vi "io_query_long_data.vi"(4 "Simulation read buffer (\"Simulation\")":string="Simulation", 6 "Block Logging (F)":bool, 8 "error in":errorcluster, 9 "Max chunk read bytes count (65536)":u32=65536, 10 "write buffer":string, 11 "VISA resource name":refnum<visa-resource-name>) -> (0 "error out":errorcluster, 2 "read buffer":string, 3 "VISA resource name out":refnum<visa-resource-name>)   [LabVIEW 2014, in "rszvl_rsidr_core.lvlib"]
uses:
  rszvl_rsidr_core.lvlib
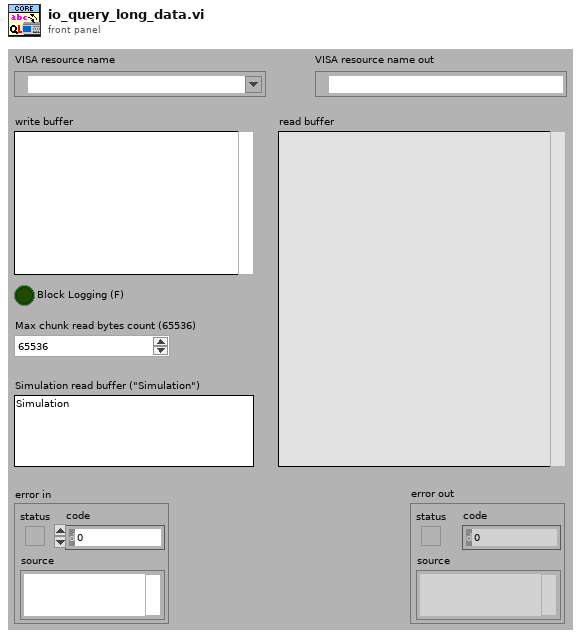
[diagram p1: front panel]
types:
  T1 = typedef "rszvl_rsidr_core.lvlib/type_Session_Data.ctl" = cluster{"Instr type":string, "Instr type for err. msg.":string, "Installed Options":string[], "OPC Timeout":i32, "Query Instrument Status":bool, "Check Range":bool, "Check Options":bool, "Add LF to Write":bool, "Simulate":bool, "Logging":bool, "Logging params":variant, "Interface Type":enum16{"Unknown", "GPIB", "VXI", "GPIB_VXI", "ASRL", "PXI", "TCPIP", "USB", "SOCKET"}, "Fast Sweep":i32, "AdditionalFlags":i32, "WaitBeforeWrite":i32, "WaitBeforeRead":i32, "BinDataChunkSize":i64}
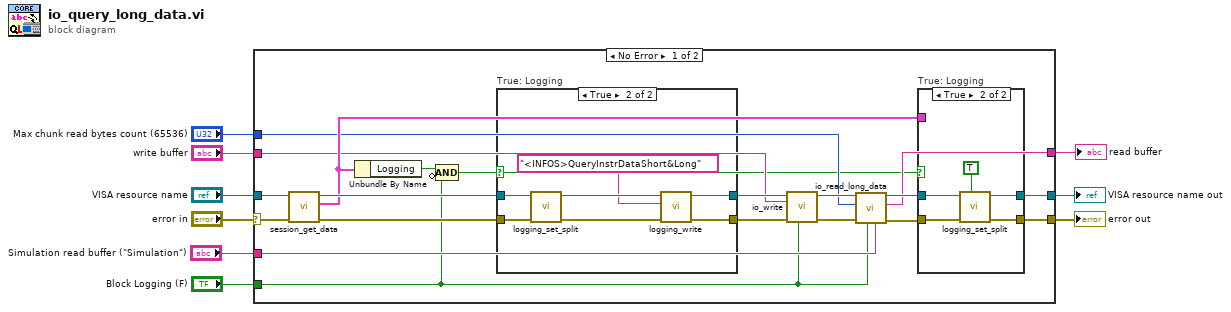
[diagram p0: block diagram]
diagram:
  n1 = case shown="No Error" "error in" {
    selector: "error in" -> [w19 w47]
    tunnel: [w13 w46] -> w3
    tunnel: [w14 w47] -> w2
    tunnel: "write buffer" -> [w16 _]
    tunnel: "VISA resource name" -> [w20 w46]
    tunnel: "Max chunk read bytes count (65536)" -> [w15 _]
    tunnel: "Simulation read buffer (\"Simulation\")" -> [w17 _]
    tunnel: [w18 _] -> w4
    tunnel: "Block Logging (F)" -> [w11 _]
    frame No Error {
      n2 = call "session_get_data.vi"("error in"=w19, "VISA resource name"=w20) -> ("error out"=w25:errorcluster, "Session User Data out"=w21:T1, "VISA resource name out"=w24:refnum<visa-resource-name>)  [unwired: 7 in]
      n3 = Unbundle By Name(w21) -> ("Logging"=w10:bool)
      n4 = Compound Arithmetic op=AND(w10, invert w11) -> (w12:bool)
      n5 = case "True: Logging" shown="True" w12 {
        tunnel: w25 -> [w38 w43]
        tunnel: w24 -> [w37 w42]
        tunnel: [w38 w45] -> w26
        tunnel: [w37 w44] -> w27
        frame False {
        }
        frame True {
          n6 = call "logging_set_split.vi"("error in"=w43, "VISA resource name"=w42) -> ("error out"=w41:errorcluster, "VISA resource name out"=w40:refnum<visa-resource-name>)  [unwired: 8 in]
          n7 = call "logging_write.vi"("error in"=w41, "String to write"="<INFOS>QueryInstrDataShort&Long" ("format string"), "VISA resource name"=w40) -> ("error out"=w45:errorcluster, "VISA resource name out"=w44:refnum<visa-resource-name>)  [unwired: 7 in]
        }
      }
      n8 = call "io_write.vi"("Block Logging (F)"=w11, "error in"=w26, "write buffer"=w16, "VISA resource name"=w27) -> ("error out"=w28:errorcluster, "VISA resource name out"=w29:refnum<visa-resource-name>)  [unwired: 6 in]
      n9 = call "io_read_long_data.vi"("Simulation read buffer (\"Simulation\")"=w17, "Block Logging (F)"=w11, "error in"=w28, "Max chunk read bytes count (65536)"=w15, "VISA resource name"=w29) -> ("error out"=w23:errorcluster, "read buffer"=w18:string, "VISA resource name out"=w22:refnum<visa-resource-name>)  [unwired: 3 in, 1 out]
      n10 = case "True: Logging" shown="True" w12 {
        tunnel: w23 -> [w31 w36]
        tunnel: [w31 w34] -> w14
        tunnel: w22 -> [w30 w35]
        tunnel: [w30 w33] -> w13
        tunnel: w21 -> [_ _]
        frame False {
        }
        frame True {
          n11 = call "logging_set_split.vi"("Evaluate section error (F)"=TRUE, "error in"=w36, "VISA resource name"=w35) -> ("error out"=w34:errorcluster, "VISA resource name out"=w33:refnum<visa-resource-name>)  [unwired: 7 in]
        }
      }
    }
    frame Error {
    }
  }
  "VISA resource name out" <- w3
  "error out" <- w2
  "read buffer" <- w4
